vi "NewController.vi"(8 "error in (no error)":errorcluster, 10 "Controls":T1) -> (0 "error out":errorcluster, 3 "Panel_UI out":refnum<class "Panel_UI.lvclass">)   [LabVIEW 2015, in "Panel_UI.lvclass"]
uses:
  Panel_UI.lvclass
  TypeDefine/MainCtlsAndVIRef.ctl
  Panel_UI.lvclass/Panel_UI.ctl
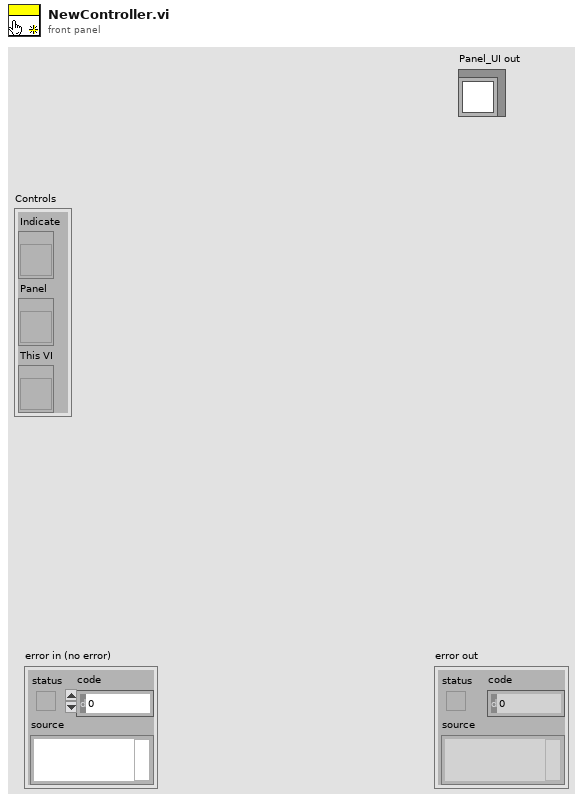
[diagram p1: front panel]
types:
  T1 = typedef "MainCtlsAndVIRef.ctl" = cluster{"Indicate":refnum<vi>, "Panel":refnum<vi>, "This VI":refnum<vi>}
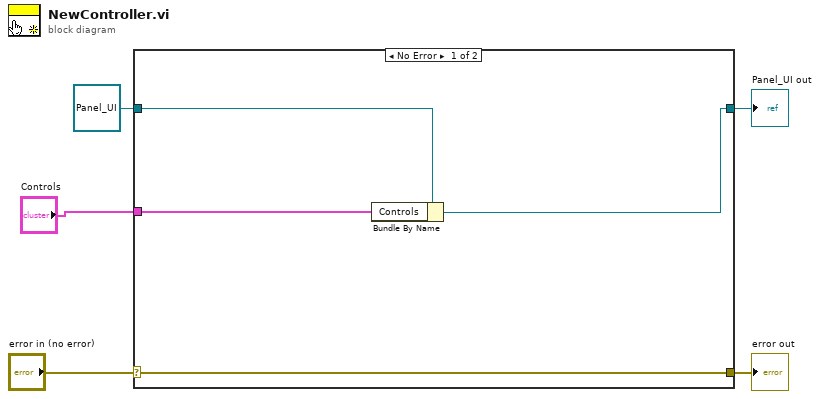
[diagram p0: block diagram]
diagram:
  n1 = case shown="No Error" "error in (no error)" {
    selector: "error in (no error)" -> [w9 w11]
    tunnel: [w9 w11] -> w4
    tunnel: [w6 w10] -> w2
    tunnel: refnum<class "Panel_UI.lvclass"> refnum ("Panel_UI in") -> [w8 w10]
    tunnel: "Controls" -> [w7 _]
    frame No Error {
      n2 = Bundle By Name(cluster=w8, "Controls"=w7) -> (w6:refnum<class "Panel_UI.lvclass">)
    }
    frame Error {
    }
  }
  "error out" <- w4
  "Panel_UI out" <- w2
